vi "Write State Machine.lvclass.vi"(8 "error in (no error)":errorcluster, 10 "State Machine.lvclass":refnum<class "State Machine.lvclass">, 11 "NewSocket in":refnum<class "NewSocket.lvclass">) -> (0 "error out":errorcluster, 3 "NewSocket out":refnum<class "NewSocket.lvclass">)   [LabVIEW 2018, in "NewSocket.lvclass"]
uses:
  NewSocket.lvclass
  State Machine/State Machine.lvclass
  NewSocket.lvclass/NewSocket.ctl
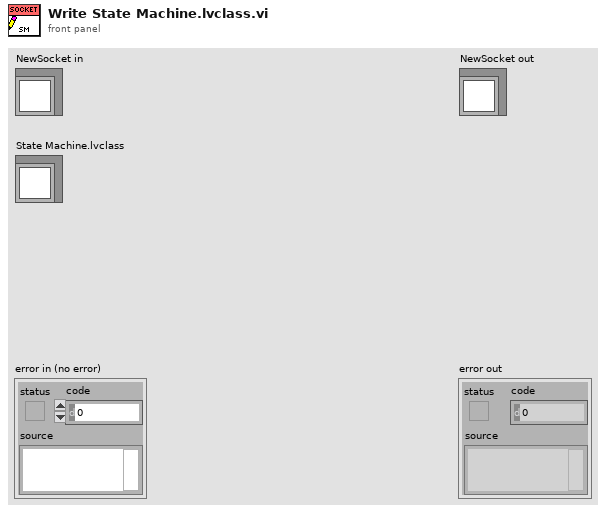
[diagram p1: front panel]
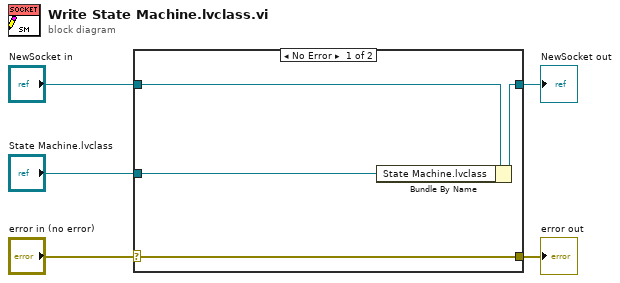
[diagram p0: block diagram]
diagram:
  n1 = case shown="No Error" "error in (no error)" {
    selector: "error in (no error)" -> [w9 w10]
    tunnel: [w9 w10] -> w4
    tunnel: [w7 w11] -> w2
    tunnel: "NewSocket in" -> [w8 w11]
    tunnel: "State Machine.lvclass" -> [w6 _]
    frame No Error {
      n2 = Bundle By Name(cluster=w8, "State Machine.lvclass"=w6) -> (w7:refnum<class "NewSocket.lvclass">)
    }
    frame Error {
    }
  }
  "error out" <- w4
  "NewSocket out" <- w2
